vi "EV Rotator Control Disengage Motors.vi"(0 "Run Step Inputs":T1={"Data in"=[], "Results in"=[], "Seq Setup in"="", "Step name"="", "Hardware in"="", "Calibration in"="", "Step # in sequence"=0, "Display step?(f)"=TRUE, "Generate names only"=FALSE, "Waveforms in"=[], "Memory List Grouping info"=[]} {"Waveforms in"."Y dB ref" format="%.1f"; "Waveforms in"."Y axis" items=["dB", "Lin", "Pwr"]; "Waveforms in"."Y data" items=["dB", "Lin", "Pwr"]; "Waveforms in"."X data" items=["dB", "Lin", "Pwr"]; "Data in"."Z data" items=["dB", "Lin", "Pwr"]; "Data in"."X data" items=["dB", "Lin", "Pwr"]; "Data in"."Y data" items=["dB", "Lin", "Pwr"]; "Data in"."Z dB ref" format="%.1f"; "Data in"."Z axis" items=["Log", "Lin"]; "Data in"."X dB ref" format="%.1f"; "Data in"."X axis" items=["Log", "Lin"]; "Data in"."Y axis" items=["Log", "Lin"]; "Data in"."Y dB ref" format="%.1f"; "Data in"."Curve"."z" format="%.2f"; "Data in"."Curve"."y" format="%.2f"; "Data in"."Curve"."x" format="%.2f"; "Results in"."Unit type" items=["dB", "Lin", "Pwr"]; "Results in"."Margin" format="%.2f"}, 11 "error in (no error)":errorcluster) -> (6 "Data out":T2 {"Z data" items=["dB", "Lin", "Pwr"]; "X data" items=["dB", "Lin", "Pwr"]; "Y data" items=["dB", "Lin", "Pwr"]; "Z dB ref" format="%.1f"; "Z axis" items=["Log", "Lin"]; "X dB ref" format="%.1f"; "X axis" items=["Log", "Lin"]; "Y axis" items=["Log", "Lin"]; "Y dB ref" format="%.1f"; "Curve"."z" format="%.2f"; "Curve"."y" format="%.2f"; "Curve"."x" format="%.2f"}, 8 "Results out":T5 {"Unit type" items=["dB", "Lin", "Pwr"]; "Margin" format="%.2f"}, 10 "Waveforms out":T7 {"Y dB ref" format="%.1f"; "Y axis" items=["dB", "Lin", "Pwr"]; "Y data" items=["dB", "Lin", "Pwr"]; "X data" items=["dB", "Lin", "Pwr"]}, 15 "error out":errorcluster)   [LabVIEW 2018]
uses:
  custom and Sc run Seq Sub VIs (x64).llb/window stack manager Functions.ctl
  custom and Sc run Seq Sub VIs (x64).llb/memlist data type.ctl
  G:/AP_Testing/Emma Dufresne/rotator/Custom VIs/EV.Rotator.RotatorControl.dll
  EV.Rotator.RotatorControl.dll
  custom and Sc run Seq Sub VIs (x64).llb/data array.ctl
  custom and Sc run Seq Sub VIs (x64).llb/result cluster.ctl
  custom and Sc run Seq Sub VIs (x64).llb/result array.ctl
  custom and Sc run Seq Sub VIs (x64).llb/waveform array.ctl
  custom and Sc run Seq Sub VIs (x64).llb/data cluster.ctl
  custom and Sc run Seq Sub VIs (x64).llb/waveform cluster.ctl
  custom and Sc run Seq Sub VIs (x64).llb/Axis Unit Type.ctl
  custom and Sc run Seq Sub VIs (x64).llb/Run Step Inputs.ctl
  custom and Sc run Seq Sub VIs (x64).llb/Memory List Grouping.ctl
  custom and Sc run Seq Sub VIs (x64).llb/Memory List Grouping - Item Type.ctl
panel:
  out "Vert/mmm angle from step":dbl
  out "Horz/ppp angle from step":dbl
  out "Mmm / vert memlist out":dbl
  out "Ppp / horz memlist out":dbl
  out "Horizontal memlist in":dbl
  out "Vertical memlist in":dbl
  out "Meridian memlist in":dbl
  out "Parallel memlist in":dbl
  # "NOTE:  These controls and indicators must stay here, but you can Hide them if you wish.  These are wired as the standard input/output connector pane for step run VIs."
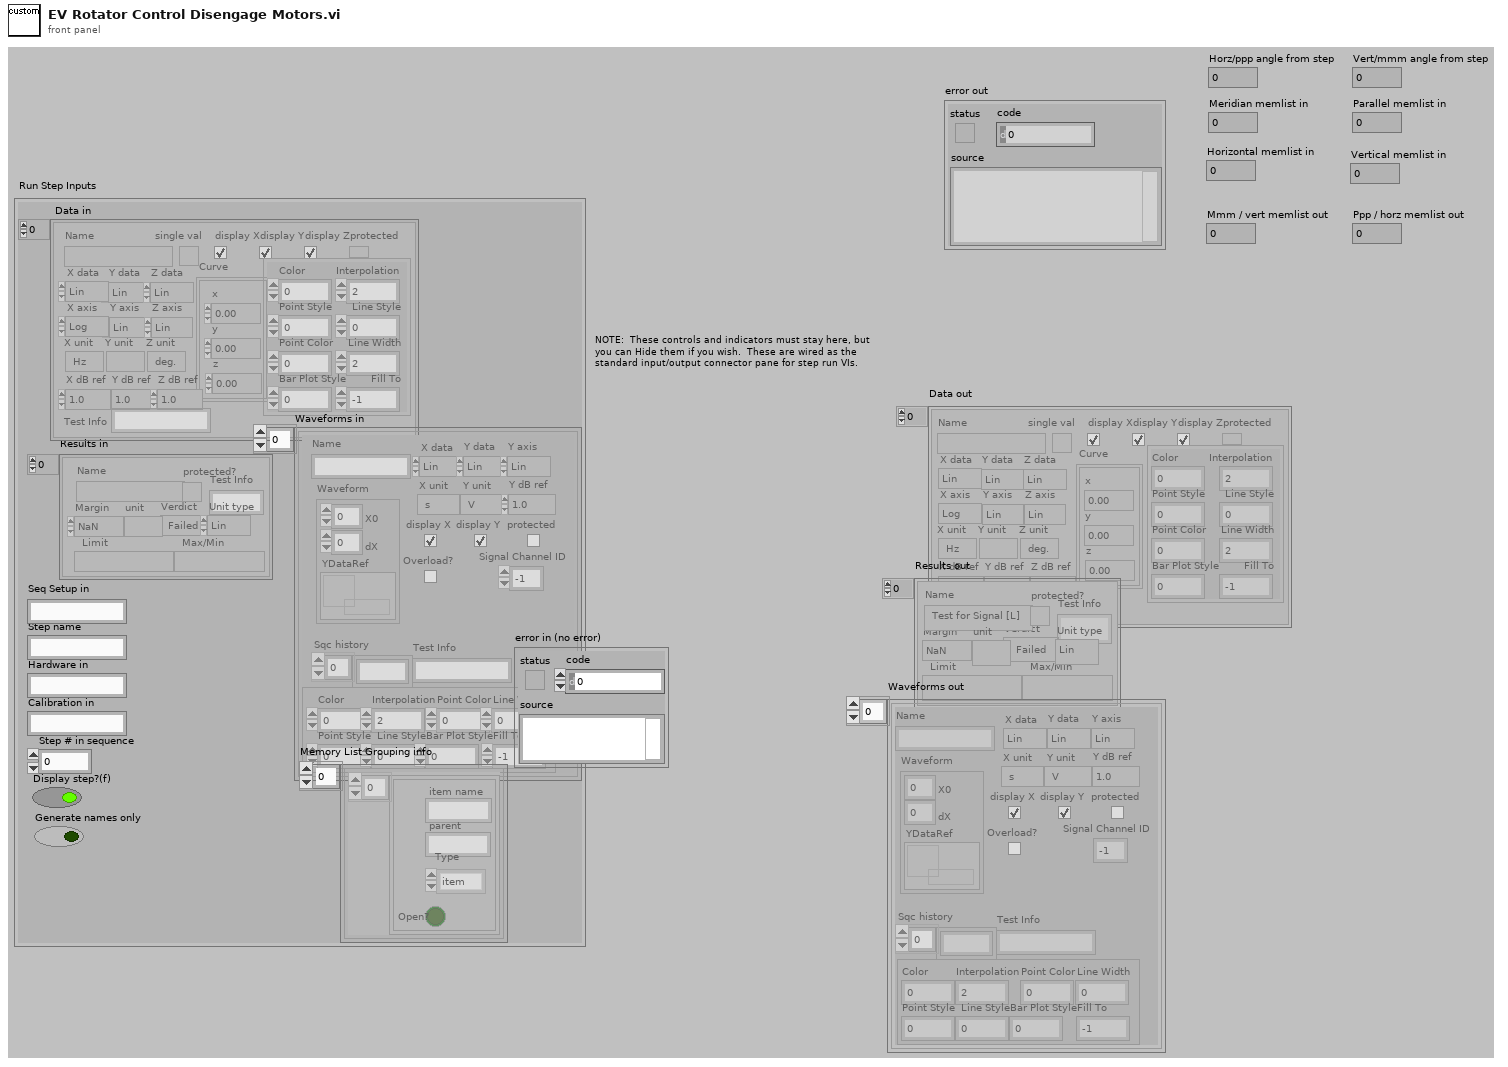
[diagram p1: front panel]
types:
  T1 = typedef "Run Step Inputs.ctl" = cluster{"Data in":T2, "Results in":T5, "Seq Setup in":string, "Step name":string, "Hardware in":string, "Calibration in":string, "Step # in sequence":i32, "Display step?(f)":bool, "Generate names only":bool, "Waveforms in":T7, "Memory List Grouping info":cluster{T9[]}[]}
  T2 = typedef "data array.ctl" = T3[]
  T3 = typedef "data cluster.ctl" = cluster{"Name":string, "Curve":cluster{"x":dbl, "y":dbl, "z":dbl}[], "X data":T4, "Y data":T4, "Z data":T4, "X axis":u16, "Y axis":u16, "Z axis":u16, "X unit":string, "Y unit":string, "Z unit":string, "X dB ref":dbl, "Y dB ref":dbl, "Z dB ref":dbl, "single val":bool, "protected":bool, "display X":bool, "display Y":bool, "display Z":bool, "Plot Settings":cluster{"Color":u32, "Interpolation":u8, "Point Style":u8, "Line Style":u8, "Point Color":u32, "Line Width":u8, "Bar Plot Style":u8, "Fill To":i16}, "Test Info":string}
  T4 = typedef "Axis Unit Type.ctl" = u16
  T5 = typedef "result array.ctl" = T6[]
  T6 = typedef "result cluster.ctl" = cluster{"Name":string, "Margin":dbl, "unit":string, "Verdict":bool, "Limit":string, "Max/Min":string, "protected?":bool, "Test Info":string, "Unit type":T4}
  T7 = typedef "waveform array.ctl" = T8[]
  T8 = typedef "waveform cluster.ctl" = cluster{"Name":string, "Waveform":cluster{"X0":dbl, "dX":dbl, "YDataRef":refnum<data-value>}, "X data":T4, "Y data":T4, "Y axis":T4, "X unit":string, "Y unit":string, "Y dB ref":dbl, "display Y":bool, "display X":bool, "Overload?":bool, "protected":bool, "Sqc history":string[], "Signal Channel ID":i32, "Plot Settings":cluster{"Color":u32, "Interpolation":u8, "Point Style":u8, "Line Style":u8, "Point Color":u32, "Line Width":u8, "Bar Plot Style":u8, "Fill To":i16}, "Test Info":string}
  T9 = typedef "Memory List Grouping.ctl" = cluster{"item name":string, "parent":string, "Open?":bool, "Type":T10}
  T10 = typedef "Memory List Grouping - Item Type.ctl" = enum16{"item", "custom group", "auto group", "protected group"}
  T11 = typedef "window stack manager Functions.ctl" = enum16{"Init", "add", "remove", "run", "clear", "vi stopped offset", "minimize all", "restore all", "autoadd", "Hourglass On", "Hourglass Off"}
  T12 = typedef "memlist data type.ctl" = enum32{"curve", "value", "result", "waveform"}
  T13 = cluster{"Horz/par angle":dbl, "Vert/mer angle":dbl, "Function to run":enum16{"MoveDegrees", "EaseToEVCoords"}, "Absolute position?":bool}
  T14 = typedef "seq step setup.ctl" = cluster{"Input Signal Channels":i32[], "Output Signal Channels":i32[], "Curves selected":string[][], "Curves generated":string[], "Step setup flat":string, "Trigger Signal Channel":i32, "Curves Generated Assumptions":cluster{"seq-setup in":string, "Relevant subset of mem list Grouping":cluster{T9[]}[]}}
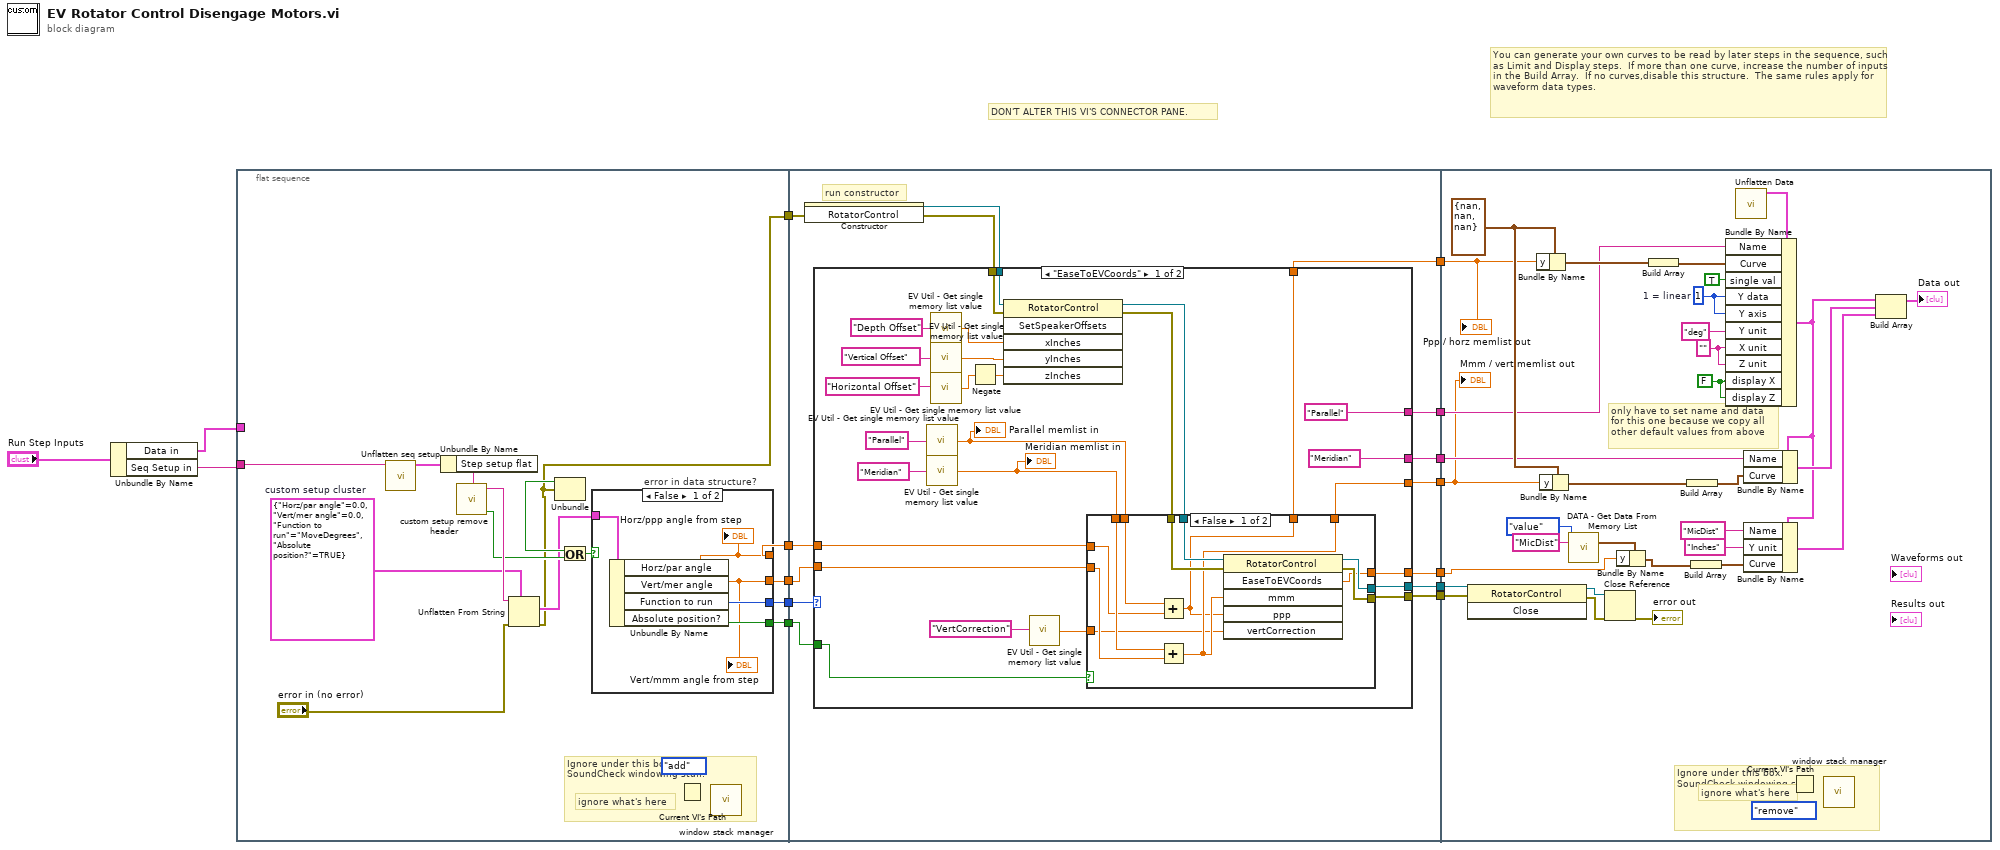
[diagram p0: block diagram]
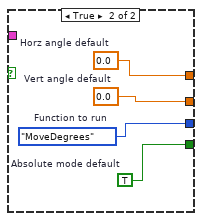
[diagram p2: hidden frame]
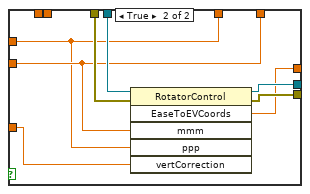
[diagram p3: hidden frame]
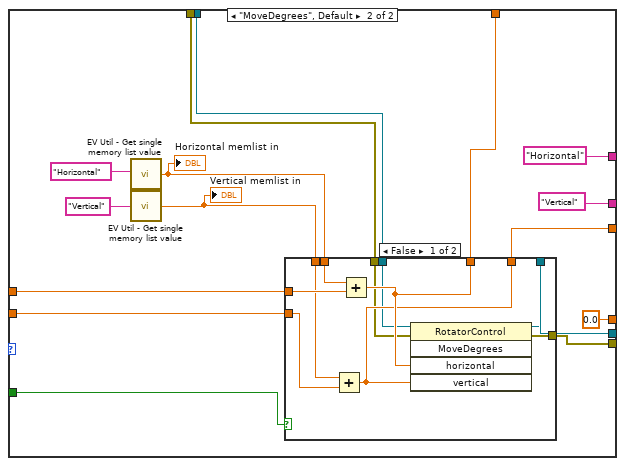
[diagram p4: hidden frame]
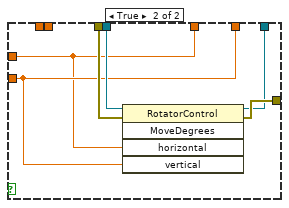
[diagram p5: hidden frame]
diagram:
  # "You can generate your own curves to be read by later steps in the sequence, such as Limit and Display steps.  If more than one curve, increase the number of inputs in the Build Array.  If no curves,disable this structure.  The same rules apply for waveform data types."
  # "DON'T ALTER THIS VI'S CONNECTOR PANE."
  n1 = Unbundle By Name("Run Step Inputs") -> ("Data in"=w6:T2, "Seq Setup in"=w5:string)
  n2 = flat-sequence {
    tunnel: w6 -> [_]
    tunnel: w5 -> [w23]
    tunnel: [w22] -> w14
    tunnel: [w18] -> w13
    tunnel: [w21] -> w12
    tunnel: [w20] -> w11
    tunnel: [w16] -> w1
    tunnel: w14 -> [w45]
    tunnel: w13 -> [w44]
    tunnel: w12 -> [w54]
    tunnel: w11 -> [w55]
    tunnel: [w46] -> w10
    tunnel: [w53] -> w9
    tunnel: [w52] -> w8
    tunnel: [w51] -> w7
    tunnel: [w50] -> w4
    tunnel: [w49] -> w3
    tunnel: [w48] -> w2
    tunnel: w1 -> [w47]
    tunnel: w10 -> [w140]
    tunnel: w9 -> [w135]
    tunnel: w8 -> [w157]
    tunnel: w7 -> [w156]
    tunnel: w4 -> [w152]
    tunnel: w3 -> [w151]
    tunnel: w2 -> [w139]
    frame #0 {
      w27 = T13 {"Horz/par angle"=0.0, "Vert/mer angle"=0.0, "Function to run"=enum."MoveDegrees", "Absolute position?"=TRUE}  # custom setup cluster
      # "Ignore under this box. \nSoundCheck windowing stuff."
      # "ignore what's here"
      n3 = call "Unflatten seq setup.vi"("Unflatten seq setup"=w23) -> ("Sequence-specific step set-up"=w32:T14)  [unwired: 3 in, 7 out]
      n4 = Unbundle By Name(w32) -> ("Step setup flat"=w31:string)
      n5 = call "custom setup remove header.vi"("Output from 'Step setup flat' of seq-setup structure"=w31) -> ("Error?"=w29:bool, "Flattened custom step setup cluster"=w30:string)  [unwired: 9 out]
      n6 = Unflatten From String(type=w27, binary string=w30, error in (no error)="error in (no error)") -> (value=w25:T13, error out=w16:errorcluster)  [unwired: 3 out]
      n7 = Unbundle(w16) -> ("status"=w28:bool)  [unwired: 2 out]
      n8 = Or(x=w28, y=w29) -> (x .or. y?=w26:bool)
      n9 = case "error in data structure?" shown="False" w26 {
        tunnel: [w37 w41] -> w21
        tunnel: [w33 w40] -> w20
        tunnel: [w36 w39] -> w18
        tunnel: w25 -> [w35 _]
        tunnel: [w34 w38] -> w22
        frame False {
          n10 = Unbundle By Name(w35) -> ("Horz/par angle"=w37:dbl, "Vert/mer angle"=w33:dbl, "Function to run"=w36:enum16{"MoveDegrees", "EaseToEVCoords"}, "Absolute position?"=w34:bool)
          "Horz/ppp angle from step" <- w37
          "Vert/mmm angle from step" <- w33
        }
        frame True {
          w39 = enum16{"MoveDegrees", "EaseToEVCoords"}."MoveDegrees"  # Function to run
          w38 = TRUE  # Absolute mode default
          w40 = 0.0  # Vert angle default
          w41 = 0.0  # Horz angle default
        }
      }
      n11 = Current VI's Path() -> (path=w24:path)
      n12 = call "window stack manager.vi"("VI path"=w24, "Function (run)"=window_stack_manager_Functions."add") -> ()  [unwired: 5 in, 5 out]
    }
    frame #1 {
      # "run constructor"
      n13 = constructor class="RotatorControl"(error in=w47) -> (reference out=w43:refnum<k24>, error out=w42:errorcluster)  [unwired: 2 in, 1 out]
      n14 = case shown="\"EaseToEVCoords\"" w44 {
        tunnel: w54 -> [w80 w115]
        tunnel: w55 -> [w79 w114]
        tunnel: w45 -> [w78 w116]
        tunnel: [w82 w113] -> w50
        tunnel: [w81 w112] -> w49
        tunnel: [w77 w111] -> w46
        tunnel: [w76 w110] -> w53
        tunnel: ["Meridian" ("Bundle Element") "Vertical" ("Bundle Element")] -> w52
        tunnel: ["Parallel" ("Bundle Element") "Horizontal" ("Bundle Element")] -> w51
        tunnel: [w73 0.0 ("EaseToEVCoords")] -> w48
        tunnel: w43 -> [w57 w103]
        tunnel: w42 -> [w56 w104]
        frame "EaseToEVCoords" {
          n15 = call "EV Util - Get single memory list value.vi"("Memory list value name"="Parallel" ("Curve name desired")) -> ("Output single value"=w68:dbl)
          "Parallel memlist in" <- w68
          n16 = call "EV Util - Get single memory list value.vi"("Memory list value name"="Meridian" ("Curve name desired")) -> ("Output single value"=w67:dbl)
          "Meridian memlist in" <- w67
          n17 = call "EV Util - Get single memory list value.vi"("Memory list value name"="Depth Offset" ("Curve name desired")) -> ("Output single value"=w60:dbl)
          n18 = call "EV Util - Get single memory list value.vi"("Memory list value name"="Vertical Offset" ("Curve name desired")) -> ("Output single value"=w62:dbl)
          n19 = call "EV Util - Get single memory list value.vi"("Memory list value name"="Horizontal Offset" ("Curve name desired")) -> ("Output single value"=w64:dbl)
          n20 = Negate(x=w64) -> (-x=w66:dbl)
          n21 = invoke class="RotatorControl" method="SetSpeakerOffsets"(reference=w57, error in=w56, "xInches"=w60, "yInches"=w62, "zInches"=w66) -> (reference out=w58:refnum<k24>, error out=w59:errorcluster)  [unwired: 1 in, 4 out]
          n22 = call "EV Util - Get single memory list value.vi"("Memory list value name"="VertCorrection" ("Curve name desired")) -> ("Output single value"=w71:dbl)
          n23 = case shown="False" w78 {
            tunnel: w58 -> [w88 w102]
            tunnel: w59 -> [w87 w101]
            tunnel: [w93 w100] -> w82
            tunnel: [w94 w99] -> w81
            tunnel: w80 -> [w90 w97]
            tunnel: w79 -> [w92 w98]
            tunnel: [w85 w97] -> w77
            tunnel: [w86 w98] -> w76
            tunnel: w68 -> [w89 _]
            tunnel: w67 -> [w91 _]
            tunnel: [w84 w96] -> w73
            tunnel: w71 -> [w83 w95]
            frame False {
              n24 = Add(x=w89, y=w90) -> (x+y=w85:dbl)
              n25 = Add(x=w91, y=w92) -> (x+y=w86:dbl)
              n26 = invoke class="RotatorControl" method="EaseToEVCoords"(reference=w88, error in=w87, "mmm"=w86, "ppp"=w85, "vertCorrection"=w83) -> (reference out=w94:refnum<k24>, error out=w93:errorcluster, "EaseToEVCoords"=w84:dbl)  [unwired: 1 in, 3 out]
            }
            frame True {
              n27 = invoke class="RotatorControl" method="EaseToEVCoords"(reference=w102, error in=w101, "mmm"=w98, "ppp"=w97, "vertCorrection"=w95) -> (reference out=w99:refnum<k24>, error out=w100:errorcluster, "EaseToEVCoords"=w96:dbl)  [unwired: 1 in, 3 out]
            }
          }
        }
        frame "MoveDegrees", Default {
          n28 = call "EV Util - Get single memory list value.vi"("Memory list value name"="Horizontal" ("Curve name desired")) -> ("Output single value"=w106:dbl)
          "Horizontal memlist in" <- w106
          n29 = call "EV Util - Get single memory list value.vi"("Memory list value name"="Vertical" ("Curve name desired")) -> ("Output single value"=w105:dbl)
          "Vertical memlist in" <- w105
          n30 = case shown="False" w116 {
            tunnel: w115 -> [w125 w129]
            tunnel: w114 -> [w123 w130]
            tunnel: [w128 w134] -> w113
            tunnel: [w127 w133] -> w112
            tunnel: w104 -> [w120 w132]
            tunnel: w103 -> [w119 w131]
            tunnel: w106 -> [w126 _]
            tunnel: w105 -> [w124 _]
            tunnel: [w122 w129] -> w111
            tunnel: [w121 w130] -> w110
            frame False {
              n31 = Add(x=w124, y=w123) -> (x+y=w121:dbl)
              n32 = Add(x=w126, y=w125) -> (x+y=w122:dbl)
              n33 = invoke class="RotatorControl" method="MoveDegrees"(reference=w119, error in=w120, "horizontal"=w122, "vertical"=w121) -> (reference out=w127:refnum<k24>, error out=w128:errorcluster)  [unwired: 1 in, 3 out]
            }
            frame True {
              n34 = invoke class="RotatorControl" method="MoveDegrees"(reference=w131, error in=w132, "horizontal"=w129, "vertical"=w130) -> (reference out=w133:refnum<k24>, error out=w134:errorcluster)  [unwired: 1 in, 3 out]
            }
          }
        }
      }
    }
    frame #2 {
      w136 = "" ("X unit")
      w137 = FALSE ("display X")
      w158 = cluster{"x":dbl, "y":dbl, "z":dbl} {"x"=nan, "y"=nan, "z"=nan}
      w161 = u16 1  # 1 = linear
      # "Ignore under this box. \nSoundCheck windowing stuff."
      # "only have to set name and data\nfor this one because we copy all\nother default values from above"
      # "ignore what's here"
      n35 = invoke class="RotatorControl" method="Close"(reference=w151, error in=w152) -> (reference out=w142:refnum<k24>, error out=w143:errorcluster)  [unwired: 1 in, 1 out]
      n36 = Bundle By Name(cluster=w158, "y"=w140) -> (w165:cluster{"x":dbl, "y":dbl, "z":dbl})
      n37 = Bundle By Name(cluster=w158, "y"=w135) -> (w160:cluster{"x":dbl, "y":dbl, "z":dbl})
      n38 = call "DATA - Get Data From Memory List.vi"("Data type"=memlist_data_type."value", "Data Name"="MicDist") -> ("value"=w150:cluster{"x":dbl, "y":dbl, "z":dbl})  [unwired: 7 in, 6 out]
      n39 = Close Reference(reference=w142, error in (no error)=w143) -> (error out=→"error out":errorcluster)
      n40 = Bundle By Name(cluster=w150, "y"=w139) -> (w144:cluster{"x":dbl, "y":dbl, "z":dbl})
      n41 = Build Array(w165) -> (w164:cluster{"x":dbl, "y":dbl, "z":dbl}[])
      n42 = Build Array(w160) -> (w159:cluster{"x":dbl, "y":dbl, "z":dbl}[])
      n43 = Build Array(w144) -> (w145:cluster{"x":dbl, "y":dbl, "z":dbl}[])
      n44 = call "Unflatten Data.vi"() -> ("Datum"=w166:T3)  [unwired: 1 in, 10 out]
      n45 = Bundle By Name(cluster=w166, "Name"=w156, "Curve"=w164, "single val"=TRUE ("T = data is just a single number (the Y element)"), "Y data"=w161, "Y axis"=w161, "Y unit"="deg" ("X unit"), "X unit"=w136, "Z unit"=w136, "display X"=w137, "display Z"=w137) -> (w147:T3)
      n46 = Bundle By Name(cluster=w147, "Name"=w157, "Curve"=w159) -> (w155:T3)
      n47 = Bundle By Name(cluster=w147, "Name"="MicDist", "Y unit"="Inches" ("X unit"), "Curve"=w145) -> (w146:T3)
      n48 = Current VI's Path() -> (path=w167:path)
      n49 = call "window stack manager.vi"("VI path"=w167, "Function (run)"=window_stack_manager_Functions."remove") -> ()  [unwired: 5 in, 5 out]
      n50 = Build Array(w147, w155, w146) -> (→"Data out":T3[])
      "Ppp / horz memlist out" <- w140
      "Mmm / vert memlist out" <- w135
    }
  }
